vi "AddPRG.vi"(0 "Protocol in":refnum<class "Protocol.lvclass">, 1 "New PRG":refnum<class "Program.lvclass">, 3 "error in (no error)":errorcluster) -> (7 "Protocol out":refnum<class "Protocol.lvclass">, 10 "error out":errorcluster)   [LabVIEW 2012, in "Protocol.lvclass"]
uses:
  Protocol.lvclass
  PRG/Program.lvclass
  Protocol.lvclass/Protocol.ctl
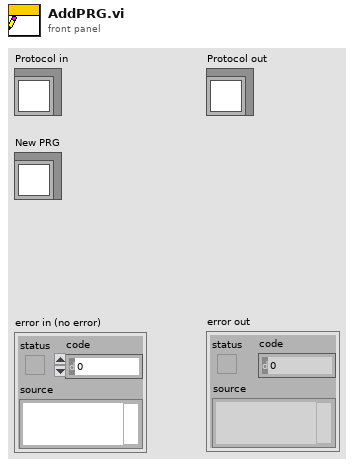
[diagram p1: front panel]
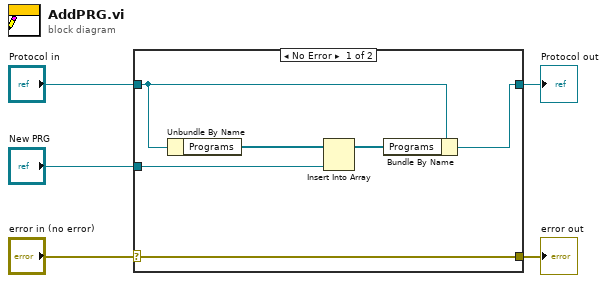
[diagram p0: block diagram]
diagram:
  n1 = case shown="No Error" "error in (no error)" {
    selector: "error in (no error)" -> [w11 w12]
    tunnel: [w11 w12] -> w4
    tunnel: [w10 w13] -> w2
    tunnel: "Protocol in" -> [w9 w13]
    tunnel: "New PRG" -> [w6 _]
    frame No Error {
      n2 = Unbundle By Name(w9) -> ("Programs"=w8:refnum<class "Program.lvclass">[])
      n3 = Insert Into Array(array=w8, new element=w6) -> (w7:refnum<class "Program.lvclass">[])  [unwired: 1 in]
      n4 = Bundle By Name(cluster=w9, "Programs"=w7) -> (w10:refnum<class "Protocol.lvclass">)
    }
    frame Error {
    }
  }
  "error out" <- w4
  "Protocol out" <- w2
